vi "TDMS Reader.vi"() -> ()   [LabVIEW 2017]
panel:
  in  "Data Set":u16(ring) items=["Time Data", "Power Spectrum"]
  out "Waveform Graph":waveform(dbl)(graph)
  out "Time of Test":timestamp=timestamp(-9593226000 s since 1904-01-01)
  out "Test Operator":string
  in  "Serial Number":string
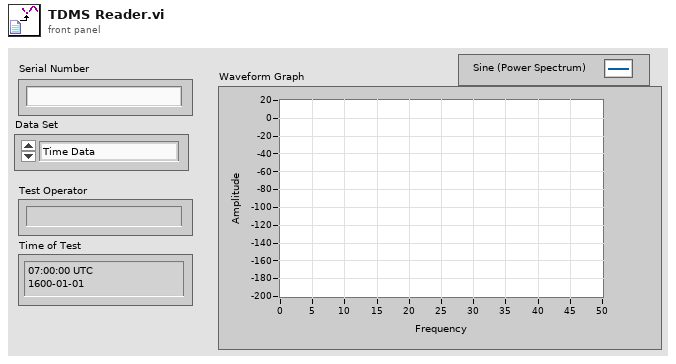
[diagram p1: front panel]
types:
  T1 = enum16{"open", "open or create", "create or replace", "create", "open (read-only)"}
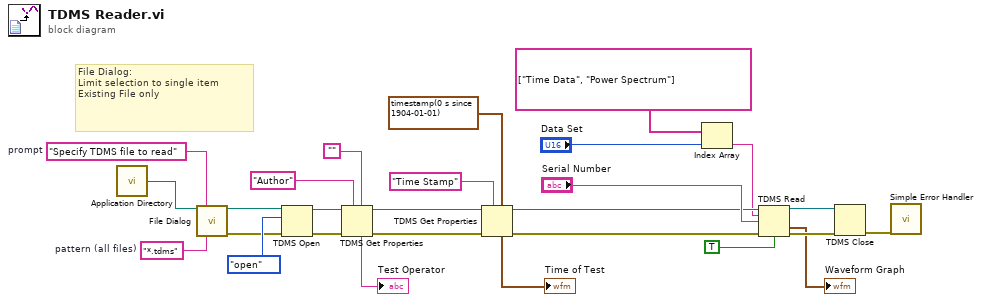
[diagram p0: block diagram]
diagram:
  w4 = "*.tdms"  # pattern (all files)
  w8 = "Specify TDMS file to read"  # prompt
  # "File Dialog:\nLimit selection to single item\nExisting File only"
  n1 = call <vilib>:"Application Directory.vi"() -> ("Application Directory"=w7:path)
  n2 = call "File Dialog"("start path"=w7, "prompt"=w8, "pattern (all files)"=w4) -> ("selected path"=w5:path, "error out"=w6:errorcluster)  [unwired: 9 in, 2 out]
  n3 = TDMS Open(8:w6, 10:T1."open" ("operation (0:open)"), 11:w5) -> (0:w22:errorcluster, 3:w23:refnum<k34>)  [unwired: 4 in]
  n4 = TDMS Get Properties(5:"", 7:"Author" ("property name"), 8:w22, 11:w23) -> (0:w19:errorcluster, 3:w21:refnum<k34>, 4:→"Test Operator":string)  [unwired: 5 out]
  n5 = TDMS Get Properties(5:timestamp(0 s since 1904-01-01), 7:"Time Stamp" ("property name"), 8:w19, 11:w21) -> (0:w18:errorcluster, 3:w20:refnum<k34>, 4:→"Time of Test":timestamp)  [unwired: 5 out]
  n6 = Index Array(array=string[] ["Time Data", "Power Spectrum"], index="Data Set") -> (element=w1:string)
  n7 = TDMS Read(0:w20, 5:w1, 7:"Serial Number", 11:w18, 13:TRUE ("return channels in file order? (F)")) -> (4:w25:refnum<k34>, 10:→"Waveform Graph":waveform(dbl), 15:w11:errorcluster)  [unwired: 3 in, 3 out]
  n8 = TDMS Close(8:w11, 11:w25) -> (0:w24:errorcluster)  [unwired: 1 out]
  n9 = call <vilib>:"Simple Error Handler.vi"("error in (no error)"=w24) -> ()  [unwired: 1 in, 8 out]
